vi "Train ramp.vi"(7 "pwr supply in":refnum<class "Power Supply.lvclass">, 9 "input":dbl[unit], 11 "field":dbl[unit]) -> (0 "output":dbl[unit], 2 "change?":bool, 3 "pwr supply out":refnum<class "Power Supply.lvclass">)   [LabVIEW 2023, in "Power Supply.lvclass"]
uses:
  Power Supply.lvclass
  Power Supply.lvclass/Power Supply.ctl
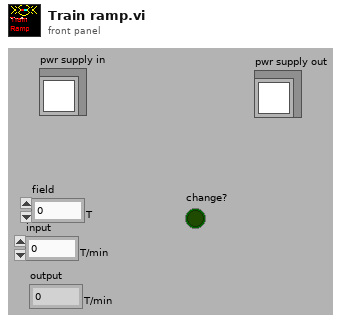
[diagram p1: front panel]
types:
  T1 = cluster{"Training Field":dbl[unit][], "Training Speed":dbl[unit][]}
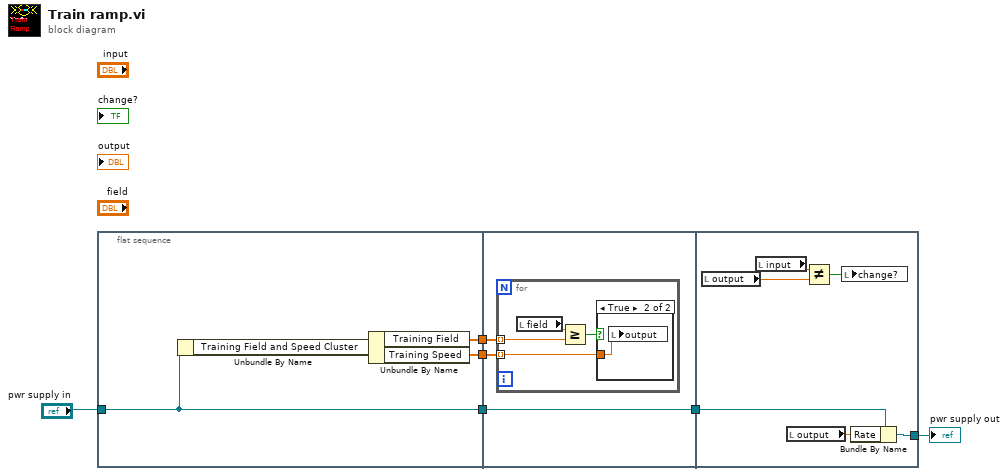
[diagram p0: block diagram]
diagram:
  n1 = flat-sequence {
    tunnel: [w9] -> w6
    tunnel: [w8] -> w5
    tunnel: [w7] -> w4
    tunnel: "pwr supply in" -> [w7]
    tunnel: w6 -> [w13]
    tunnel: w5 -> [w12]
    tunnel: w4 -> [w11]
    tunnel: [w11] -> w3
    tunnel: w3 -> [w24]
    tunnel: [w22] -> w2
    frame #0 {
      n2 = Unbundle By Name(w7) -> ("Training Field and Speed Cluster"=w10:T1)
      n3 = Unbundle By Name(w10) -> ("Training Field"=w9:dbl[unit][], "Training Speed"=w8:dbl[unit][])
    }
    frame #1 {
      n4 = for {
        tunnel: w13 -> [w16] mode=indexing
        tunnel: w12 -> [w14] mode=indexing
        n5 = local read "field"() -> (w17:dbl[unit])
        n6 = Greater Or Equal?(x=w17, y=w16) -> (x >= y?=w15:bool)
        n7 = case shown="True" w15 {
          tunnel: w14 -> [_ w18]
          frame False {
          }
          frame True {
            n8 = local write "output"(w18) -> ()
          }
        }
      }
    }
    frame #2 {
      n9 = local read "output"() -> (w20:dbl[unit])
      n10 = local read "input"() -> (w21:dbl[unit])
      n11 = local read "output"() -> (w23:dbl[unit])
      n12 = Not Equal?(x=w21, y=w20) -> (x != y?=w19:bool)
      n13 = local write "change?"(w19) -> ()
      n14 = Bundle By Name(cluster=w24, "Rate"=w23) -> (w22:refnum<class "Power Supply.lvclass">)
    }
  }
  "pwr supply out" <- w2
